vi "RunOperation.vi"(10 "Inputs":string[](array[string]), 11 "VIPMInstallPackageFile in":refnum<class "VIPMInstallPackageFile.lvclass">) -> (1 "Output/Failure":string, 2 "CLI Process Return Code":i32, 3 "VIPMInstallPackageFile out":refnum<class "VIPMInstallPackageFile.lvclass">)   [LabVIEW 2014, in "VIPMInstallPackageFile.lvclass"]
uses:
  <nishared>/LabVIEW CLI/Operations/VIPMInstallPackageFile/VIPMInstallPackageFile.lvclass
  <nishared>/LabVIEW CLI/Operations/VIPMInstallPackageFile/VIPMInstallPackageFile.lvclass/VIPMInstallPackageFile.ctl
  <userlib>/_OpenG.lib/file/file.llb/Strip Path Extension - String__ogtk.vi
  <vilib>/JKI/VIPM API/VIPM API_vipm_api.lvlib
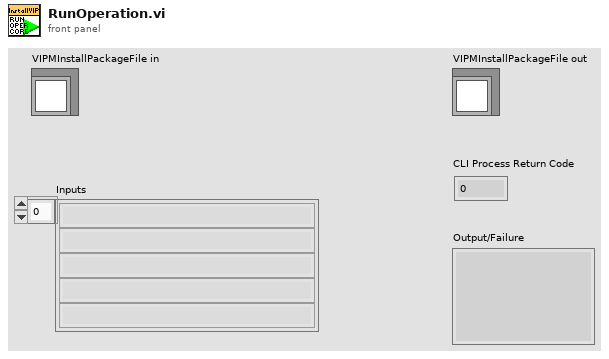
[diagram p1: front panel]
types:
  T1 = typedef "VIPM API_vipm_api.lvlib/Library Contents Cluster_vipm_api.ctl" = cluster{"Package Name":string, "Version":string, "Display Name":string, "Repository Name":string, "Company Name":string, "License Type":string, "Installed":bool, "Deprecated":bool, "Dependency or Conflict Problem":bool, "Downloaded":bool}
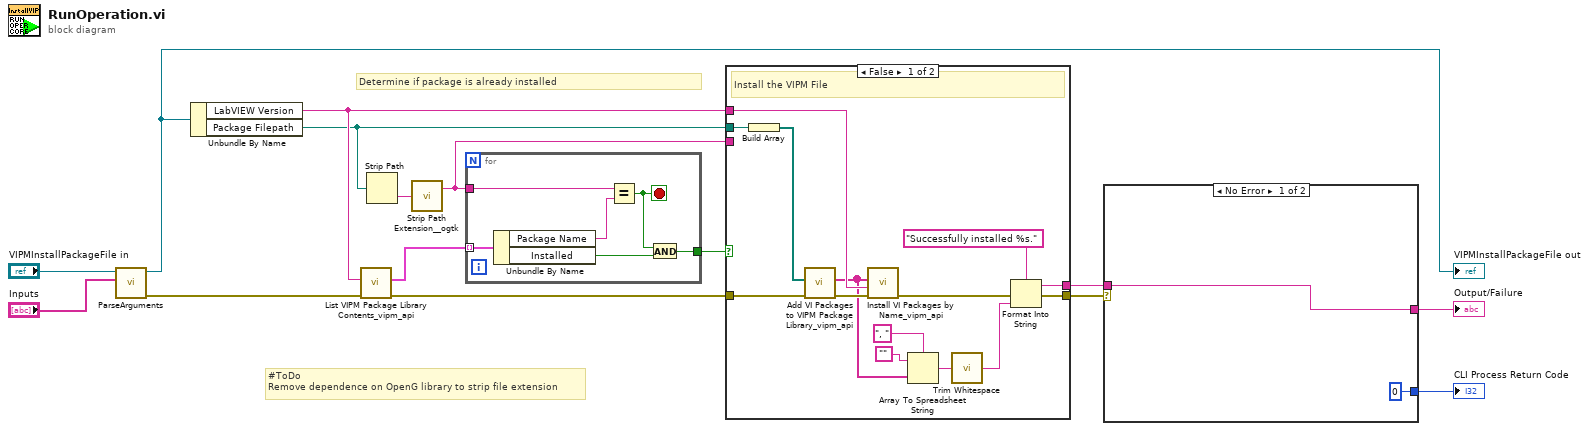
[diagram p0: block diagram]
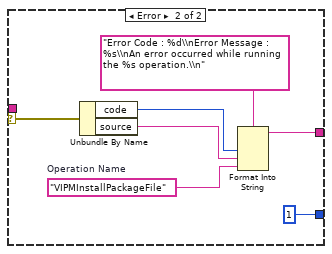
[diagram p2: hidden frame]
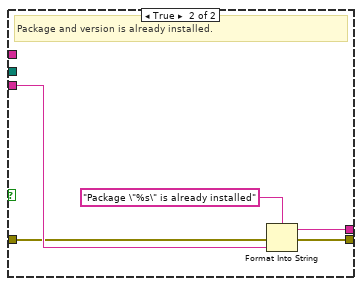
[diagram p3: hidden frame]
diagram:
  # "#ToDo\nRemove dependence on OpenG library to strip file extension"
  # "Determine if package is already installed"
  n1 = call <nishared>:"ParseArguments.vi"("Inputs"="Inputs", "VIPMInstallPackageFile in"="VIPMInstallPackageFile in") -> ("error out"=w12:errorcluster, "VIPMInstallPackageFile out"=w13:refnum<class "VIPMInstallPackageFile.lvclass">)  [unwired: 8 in]
  "VIPMInstallPackageFile out" <- w13
  n2 = Unbundle By Name(w13) -> ("LabVIEW Version"=w10:string, "Package Filepath"=w7:path)
  n3 = call <vilib>:"List VIPM Package Library Contents_vipm_api.vi"("error in (no error)"=w12, "LabVIEW Version"=w10) -> ("error out"=w11:errorcluster, "Library Contents []"=w8:T1[])  [unwired: 8 in]
  n4 = Strip Path(path=w7) -> (name=w9:string)  [unwired: 1 out]
  n5 = call-poly <userlib>:"Strip Path Extension__ogtk.vi"("path"=w9) -> ("root"=w5:string)  [unwired: 1 out]
  n6 = for {
    tunnel: w8 -> [w21] mode=indexing
    tunnel: w5 -> [w20]
    tunnel: [w16] -> w6
    stop <- w18 stop-if-true
    n7 = Unbundle By Name(w21) -> ("Package Name"=w19:string, "Installed"=w17:bool)
    n8 = Equal?(x=w20, y=w19) -> (x = y?=w18:bool)
    n9 = And(x=w18, y=w17) -> (x .and. y?=w16:bool)
  }
  n10 = case shown="False" w6 {
    tunnel: w11 -> [w33 w39]
    tunnel: w10 -> [w32 _]
    tunnel: w7 -> [w31 _]
    tunnel: w5 -> [_ w40]
    tunnel: [w23 w37] -> w2
    tunnel: [w22 w36] -> w1
    frame False {
      # "Install the VIPM File"
      n11 = Build Array(w31) -> (w34:path[])
      n12 = call <vilib>:"Add VI Packages to VIPM Package Library_vipm_api.vi"("error in (no error)"=w33, "Packages to add to VIPM Library (vipc,vip,ogp)"=w34) -> ("error out"=w35:errorcluster, "Package Names Added"=w24:string[])  [unwired: 8 in]
      n13 = call <vilib>:"Install VI Packages by Name_vipm_api.vi"("error in (no error)"=w35, "LabVIEW Version"=w32, "Package Names to Install []"=w24) -> ("error out"=w25:errorcluster)  [unwired: 8 in]
      n14 = Array To Spreadsheet String(delimiter (Tab)=", ", array=w24, 3:"") -> (spreadsheet string=w29:string)
      n15 = call <vilib>:"Trim Whitespace.vi"("string"=w29) -> ("trimmed string"=w30:string)  [unwired: 1 in]
      n16 = Format Into String(format string="Successfully installed %s.", error in=w25, w30) -> (resulting string=w22:string, error out=w23:errorcluster)  [unwired: 1 in]
    }
    frame True {
      # "Package and version is already installed."
      n17 = Format Into String(format string="Package \"%s\" is already installed", error in=w39, w40) -> (resulting string=w36:string, error out=w37:errorcluster)  [unwired: 1 in]
    }
  }
  n18 = case shown="No Error" w2 {
    selector: w2 -> [_ w49]
    tunnel: [w41 w44] -> w3
    tunnel: [0 ("CLI Process Return Code") 1 ("CLI Process Return Code")] -> w4
    tunnel: w1 -> [w41 _]
    frame No Error {
    }
    frame Error {
      w45 = "VIPMInstallPackageFile"  # Operation Name
      n19 = Unbundle By Name(w49) -> ("code"=w48:i32, "source"=w47:string)
      n20 = Format Into String(format string="Error Code : %d\\nError Message : %s\\nAn error occurred while running the %s operation.\\n" ("Format Error Output String"), w48, w47, w45) -> (resulting string=w44:string)  [unwired: 2 in, 1 out]
    }
  }
  "CLI Process Return Code" <- w4
  "Output/Failure" <- w3
